vi "ESP301_MO.vi"(10 "axisNumber":i32=1, 11 "COM_PORT":string="COM12") -> (0 "errstring":string)   [LabVIEW 2019]
uses:
  Newport.ESP301.CommandInterface
panel:
  out "MO_Set":i32
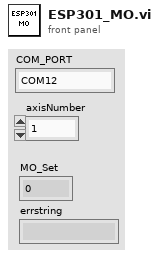
[diagram p1: front panel]
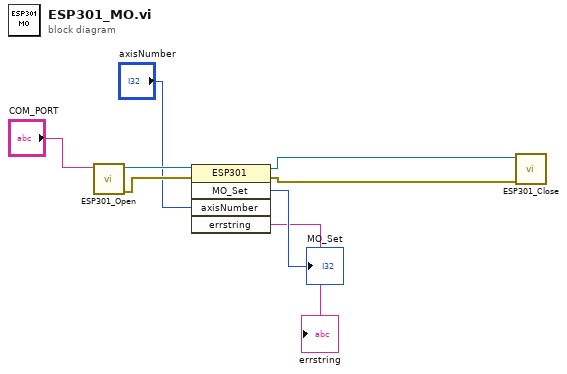
[diagram p0: block diagram]
diagram:
  n1 = call "ESP301_Open.vi"("strDeviceKey"="COM_PORT") -> ("sortie d'erreur"=w7:errorcluster, "référence en sortie"=w8:refnum<k24>)  [unwired: 9 in]
  n2 = invoke on="Nœud de méthode" class="ESP301" method="MO_Set"(reference=w8, error in=w7, "axisNumber"="axisNumber") -> (reference out=w4:refnum<k24>, error out=w3:errorcluster, "MO_Set"=→"MO_Set":i32, "errstring"=→"errstring":string)  [unwired: 2 in, 1 out]
  n3 = call "ESP301_Close.vi"("entrée d'erreur (pas d'erreur)"=w3, "référence"=w4) -> ()  [unwired: 9 in, 1 out]
